vi "NI VeriStand - Convert Timed Loop Priority to Number.vi"(11 "Priority":T1) -> (3 "Numeric Priority":i32)   [LabVIEW 2020, in "Custom Device API.lvlib"]
doc: "Converts a priority value (Low, Medium, or High) for the Timed Loop in which an asynchronous custom device runs into a numeric value that the Input node of a Timed Loop accepts. Use the NI VeriStand - Get Timed Loop Priority VI to get the priority value. You can use the NI VeriStand - Set Timed Loop Priority VI to set the priority value for a custom device Timed Loop."
uses:
  <vilib>/NI VeriStand/Custom Device API/Custom Device API.lvlib
  <vilib>/NI VeriStand/Custom Device API/Custom Device Timed Loop Priority.ctl
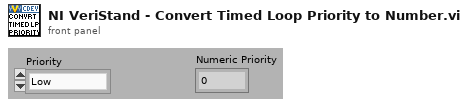
[diagram p1: front panel]
types:
  T1 = typedef "Custom Device API.lvlib/Custom Device Timed Loop Priority.ctl" = enum32{"Low", "Medium", "High"}
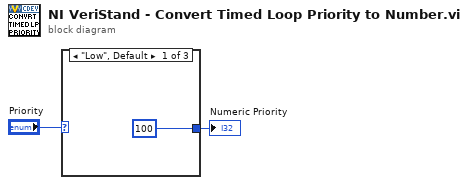
[diagram p0: block diagram]
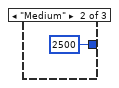
[diagram p2: hidden frame]
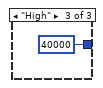
[diagram p3: hidden frame]
diagram:
  n1 = case shown="\"Low\", Default" "Priority" {
    tunnel: [100 2500 40000] -> w1
    frame "Low", Default {
    }
    frame "Medium" {
    }
    frame "High" {
    }
  }
  "Numeric Priority" <- w1
